vi "Add Device.vi"(8 "error in (no error)":errorcluster, 11 "App in":refnum<class "App.lvclass">) -> (0 "error out":errorcluster, 3 "App out":refnum<class "App.lvclass">)   [LabVIEW 2020, in "PicoG-App.lvlib" / "App.lvclass"]
uses:
  App.lvclass
  App.lvclass/App.ctl
  Builds/picoG/ppl/PicoG-Core.lvlibp/PicoG-Processor/PicoG-Core/DeployPlatform/DeployPlatform.lvclass
  Builds/picoG/ppl/PicoG-Core.lvlibp/PicoG-Processor/PicoG-Core/PlatformPluginManager/PlatformPluginManager.lvclass
  Device/Device.lvclass
  DeviceListPanel/DeviceListPanel.lvclass
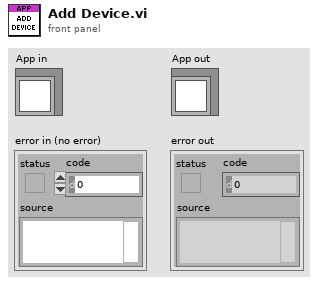
[diagram p1: front panel]
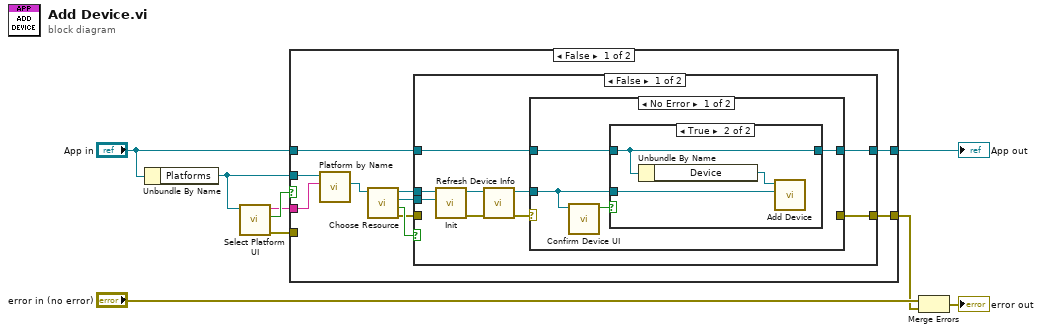
[diagram p0: block diagram]
diagram:
  n1 = Unbundle By Name("App in") -> ("Platforms"=w5:refnum<class "PlatformPluginManager.lvclass">)
  n2 = call "Select Platform UI.vi"("Plugins"=w5) -> ("error out"=w7:errorcluster, "Cancelled"=w9:bool, "Platform"=w8:string)  [unwired: 8 in]
  n3 = case shown="False" w9 {
    tunnel: w8 -> [w18 _]
    tunnel: w7 -> [_ _]
    tunnel: "App in" -> [w15 w40]
    tunnel: w5 -> [w19 _]
    tunnel: [w14 w40] -> w4
    tunnel: [w10 _] -> w1
    frame False {
      n4 = call "Platform by Name.vi"("Platform"=w18, "TargetPluginManager in"=w19) -> ("Target"=w17:refnum<class "DeployPlatform.lvclass">)  [unwired: 7 in, 2 out]
      n5 = call-dynamic "Choose Resource.vi"("DeployTarget in"=w17) -> ("error out"=w13:errorcluster, "Cancelled"=w16:bool, "Resource"=w11:refnum<class "DeployResource.lvclass">, "DeployTarget out"=w12:refnum<class "DeployPlatform.lvclass">)  [unwired: 7 in]
      n6 = case shown="False" w16 {
        tunnel: w15 -> [w24 w39]
        tunnel: [w23 w39] -> w14
        tunnel: w13 -> [_ _]
        tunnel: w12 -> [w28 _]
        tunnel: w11 -> [w27 _]
        tunnel: [w20 _] -> w10
        frame False {
          n7 = call "Init.vi"("Resource"=w27, "Platform"=w28) -> ("error out"=w25:errorcluster, "Device out"=w26:refnum<class "Device.lvclass">)  [unwired: 8 in]
          n8 = call "Refresh Device Info.vi"("error in (no error)"=w25, "Device in"=w26) -> ("error out"=w21:errorcluster, "Device out"=w22:refnum<class "Device.lvclass">)  [unwired: 8 in]
          n9 = case shown="No Error" w21 {
            selector: w21 -> [_ w38]
            tunnel: w24 -> [w31 w37]
            tunnel: [w30 w37] -> w23
            tunnel: w22 -> [w29 _]
            tunnel: [_ w38] -> w20
            frame No Error {
              n10 = call "Confirm Device UI.vi"("Device"=w29) -> ("Confirmed"=w32:bool)  [unwired: 10 in]
              n11 = case shown="True" w32 {
                tunnel: w31 -> [w33 w36]
                tunnel: [w33 w36] -> w30
                tunnel: w29 -> [_ w34]
                frame False {
                }
                frame True {
                  n12 = Unbundle By Name(w36) -> ("Device"=w35:refnum<class "DeviceListPanel.lvclass">)
                  n13 = call "Add Device.vi"("Device"=w34, "DeviceListPanel in"=w35) -> ()  [unwired: 8 in, 2 out]
                }
              }
            }
            frame Error {
            }
          }
        }
        frame True {
        }
      }
    }
    frame True {
    }
  }
  "App out" <- w4
  n14 = Merge Errors("error in (no error)", w1) -> (→"error out":errorcluster)
